vi "plot_graphs.vi"(6 "channel":i32, 8 "error in":errorcluster, 9 "angs":dbl[](array[numeric]), 10 "polar_data":T1, 11 "Plot ID":T2 format="%x") -> (0 "error out":errorcluster, 3 "Plot ID out":T2 format="%x")   [LabVIEW 2018]
uses:
  <vilib>/Heliosphere Research LLC/Advanced Plotting Toolkit/typedefs/PlotID.ctl
  polar_data.ctl
  <vilib>/Heliosphere Research LLC/Advanced Plotting Toolkit/Advanced Plotting Toolkit.lvlib
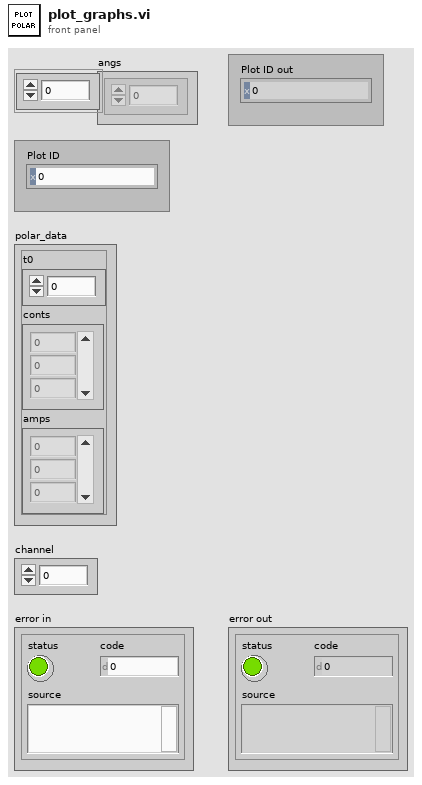
[diagram p1: front panel]
types:
  T1 = typedef "polar_data.ctl" = cluster{"t0":dbl, "conts":dbl[], "amps":dbl[]}
  T2 = typedef "Advanced Plotting Toolkit.lvlib/PlotID.ctl" = i32
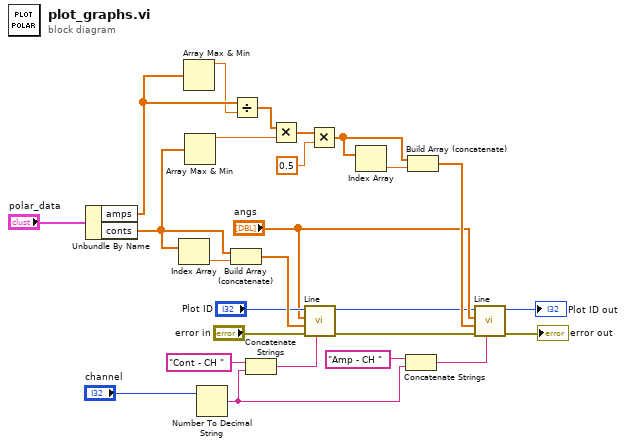
[diagram p0: block diagram]
diagram:
  n1 = Unbundle By Name("polar_data") -> ("amps"=w15:dbl[], "conts"=w13:dbl[])
  n2 = Index Array(array=w13) -> (element=w24:dbl)  [unwired: 1 in]
  n3 = Array Max & Min(array=w15) -> (max value=w14:dbl)  [unwired: 3 out]
  n4 = Array Max & Min(array=w13) -> (max value=w12:dbl)  [unwired: 3 out]
  n5 = Number To Decimal String(number="channel") -> (decimal integer string=w3:string)  [unwired: 1 in]
  n6 = Build Array (concatenate)(w13, w24) -> (w25:dbl[])
  n7 = Divide(x=w15, y=w14) -> (x/y=w11:dbl[])
  n8 = Concatenate Strings("Cont - CH " ("Legend Title"), w3) -> (w23:string)
  n9 = Multiply(x=w11, y=w12) -> (x*y=w10:dbl[])
  n10 = call <vilib>:"Line.vi"("Legend Title"=w23, "error in (no error)"="error in", "Y Data"=w25, "X Data"="angs", "Plot ID"="Plot ID") -> ("error out"=w18:errorcluster, "Plot ID out"=w1:T2)  [unwired: 5 in]
  n11 = Multiply(x=w10, y=0.5) -> (x*y=w7:dbl[])
  n12 = Index Array(array=w7) -> (element=w8:dbl)  [unwired: 1 in]
  n13 = Concatenate Strings("Amp - CH " ("Legend Title"), w3) -> (w2:string)
  n14 = Build Array (concatenate)(w7, w8) -> (w6:dbl[])
  n15 = call <vilib>:"Line.vi"("Legend Title"=w2, "error in (no error)"=w18, "Y Data"=w6, "X Data"="angs", "Plot ID"=w1) -> ("error out"=→"error out":errorcluster, "Plot ID out"=→"Plot ID out":T2)  [unwired: 5 in]
